vi "GetCleangitRevision.vi"(11 "File Path Control":path caption="File Path Control (leave blank to use Constants_Global value of EnFlo SW Folder)") -> (2 "gitDetails":string, 3 "gitRevision":string, 4 "oneLiner":string)   [LabVIEW 2022 SP3]
uses:
  <vilib>/Utility/error.llb/Trim Whitespace One-Sided.vi
  Globals/Constants_global.vi
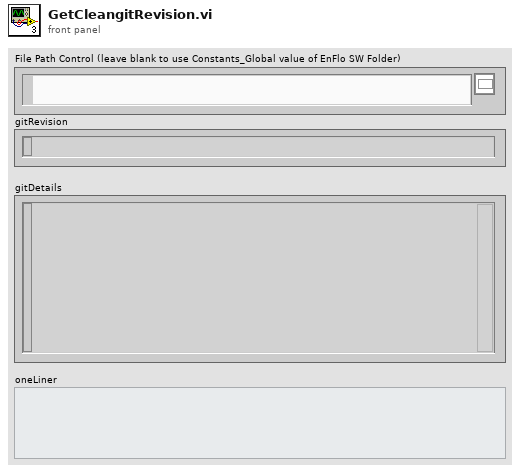
[diagram p1: front panel]
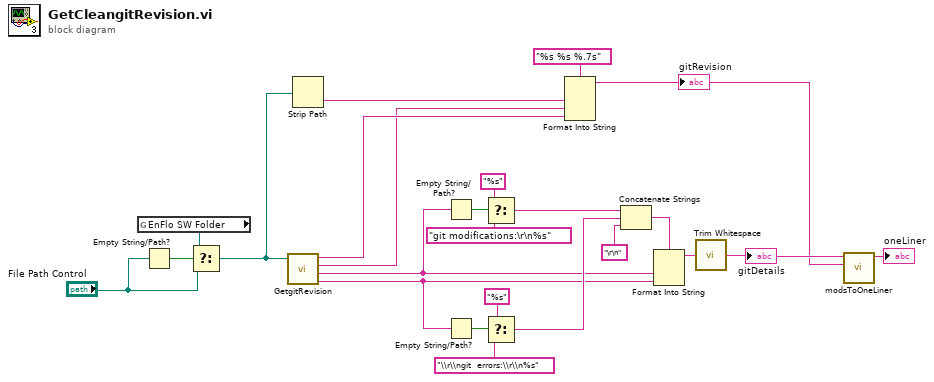
[diagram p0: block diagram]
diagram:
  n1 = global read "Constants_global.vi" "EnFlo SW Folder"() -> (w19:path)
  n2 = Empty String/Path?(string/path="File Path Control") -> (empty?=w20:bool)
  n3 = Select(t=w19, s=w20, f="File Path Control") -> (s? t:f=w17:path)
  n4 = call "GetgitRevision.vi"("File Path Control"=w17) -> ("status&log error"=w4:string, "LocalModifications"=w8:string, "branch"=w6:string, "OverallRevision"=w7:string)  [unwired: 7 in]
  n5 = Strip Path(path=w17) -> (name=w15:string)  [unwired: 1 out]
  n6 = Empty String/Path?(string/path=w8) -> (empty?=w12:bool)
  n7 = Empty String/Path?(string/path=w4) -> (empty?=w23:bool)
  n8 = Select(t="%s", s=w12, f="git modifications:\r\n%s" ("format string")) -> (s? t:f=w14:string)
  n9 = Select(t="%s" ("format string"), s=w23, f="\\r\\ngit  errors:\\r\\n%s" ("format string")) -> (s? t:f=w10:string)
  n10 = Format Into String(format string="%s %s %.7s", w15, w6, w7) -> (resulting string=w2:string)  [unwired: 2 in, 1 out]
  "gitRevision" <- w2
  n11 = Concatenate Strings(w14, w10, "\r\n" ("string")) -> (w9:string)
  n12 = Format Into String(format string=w9, w8, w4) -> (resulting string=w21:string)  [unwired: 2 in, 1 out]
  n13 = call <vilib>:"Trim Whitespace.vi"("string"=w21) -> ("trimmed string"=w3:string)  [unwired: 1 in]
  "gitDetails" <- w3
  n14 = call "modsToOneLiner.vi"("revisionNumber"=w2, "modificationLog"=w3) -> ("oneLiner"=→"oneLiner":string)  [unwired: 9 in]
